vi "KenbakFront.vi"() -> ()   [LabVIEW 2012]
panel:
  in  "Data":u8 format="%08b"
  out "Kdec":u8
  in  "Read":bool
  in  "Store":bool
  in  "AddressDec":u8
  in  "Inputs":T1
  in  "Wait (ms)":u32
  out "Instruction Specific":T2
  out "Adder":T3
  out "Clocks And Memory":T4
  out "W_reg":T5
  out "L_reg":T6
  out "T_reg":T7
  out "Mem":cluster{"MemLo":u8, "MemHi":u8, "Carry?":bool} {"MemHi" format="%x"; "MemLo" format="%x"}
  out "I_reg":T8
  out "States":T9
  out "Input":bool
  out "Run":bool
  out "Memory":bool
  out "Address":bool
  out "K_reg":T10
  out "Cycles/sec":i32
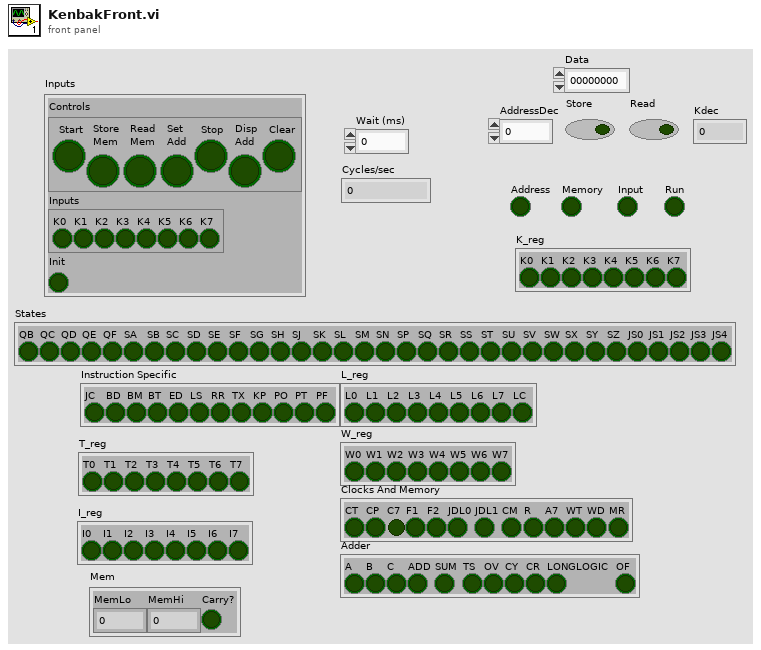
[diagram p1: front panel]
types:
  T1 = cluster{"Controls":cluster{"Start":bool, "Store\nMem":bool, "Read\nMem":bool, "Set\nAdd":bool, "Stop":bool, "Disp\nAdd":bool, "Clear":bool}, "Inputs":cluster{"K0":bool, "K1":bool, "K2":bool, "K3":bool, "K4":bool, "K5":bool, "K6":bool, "K7":bool}, "Init":bool}
  T2 = cluster{"JC":bool, "BD":bool, "BM":bool, "BT":bool, "ED":bool, "LS":bool, "RR":bool, "TX":bool, "KP":bool, "PO":bool, "PT":bool, "PF":bool}
  T3 = cluster{"A":bool, "B":bool, "C":bool, "ADD":bool, "SUM":bool, "TS":bool, "OV":bool, "CY":bool, "CR":bool, "LONGLOGIC":bool, "OF":bool}
  T4 = cluster{"CT":bool, "CP":bool, "C7":bool, "F1":bool, "F2":bool, "JDL0":bool, "JDL1":bool, "CM":bool, "R":bool, "A7":bool, "WT":bool, "WD":bool, "MR":bool}
  T5 = cluster{"W0":bool, "W1":bool, "W2":bool, "W3":bool, "W4":bool, "W5":bool, "W6":bool, "W7":bool}
  T6 = cluster{"L0":bool, "L1":bool, "L2":bool, "L3":bool, "L4":bool, "L5":bool, "L6":bool, "L7":bool, "LC":bool}
  T7 = cluster{"T0":bool, "T1":bool, "T2":bool, "T3":bool, "T4":bool, "T5":bool, "T6":bool, "T7":bool}
  T8 = cluster{"I0":bool, "I1":bool, "I2":bool, "I3":bool, "I4":bool, "I5":bool, "I6":bool, "I7":bool}
  T9 = cluster{"QB":bool, "QC":bool, "QD":bool, "QE":bool, "QF":bool, "SA":bool, "SB":bool, "SC":bool, "SD":bool, "SE":bool, "SF":bool, "SG":bool, "SH":bool, "SJ":bool, "SK":bool, "SL":bool, "SM":bool, "SN":bool, "SP":bool, "SQ":bool, "SR":bool, "SS":bool, "ST":bool, "SU":bool, "SV":bool, "SW":bool, "SX":bool, "SY":bool, "SZ":bool, "JS0":bool, "JS1":bool, "JS2":bool, "JS3":bool, "JS4":bool}
  T10 = cluster{"K0":bool, "K1":bool, "K2":bool, "K3":bool, "K4":bool, "K5":bool, "K6":bool, "K7":bool}
  T11 = cluster{"[0]":bool, "[1]":bool, "[2]":bool, "[3]":bool, "[4]":bool, "[5]":bool, "[6]":bool, "[7]":bool}
  T12 = cluster{"GO":bool, "EN":bool, "DD":bool, "EA":bool, "HT":bool, "DA":bool, "CL":bool, "ADD":bool, "MEM":bool, "RUN":bool, "INPUT":bool, "X1":bool, "X2":bool, "X3":bool, "X4":bool, "BU":bool, "KS":bool, "FT":bool}
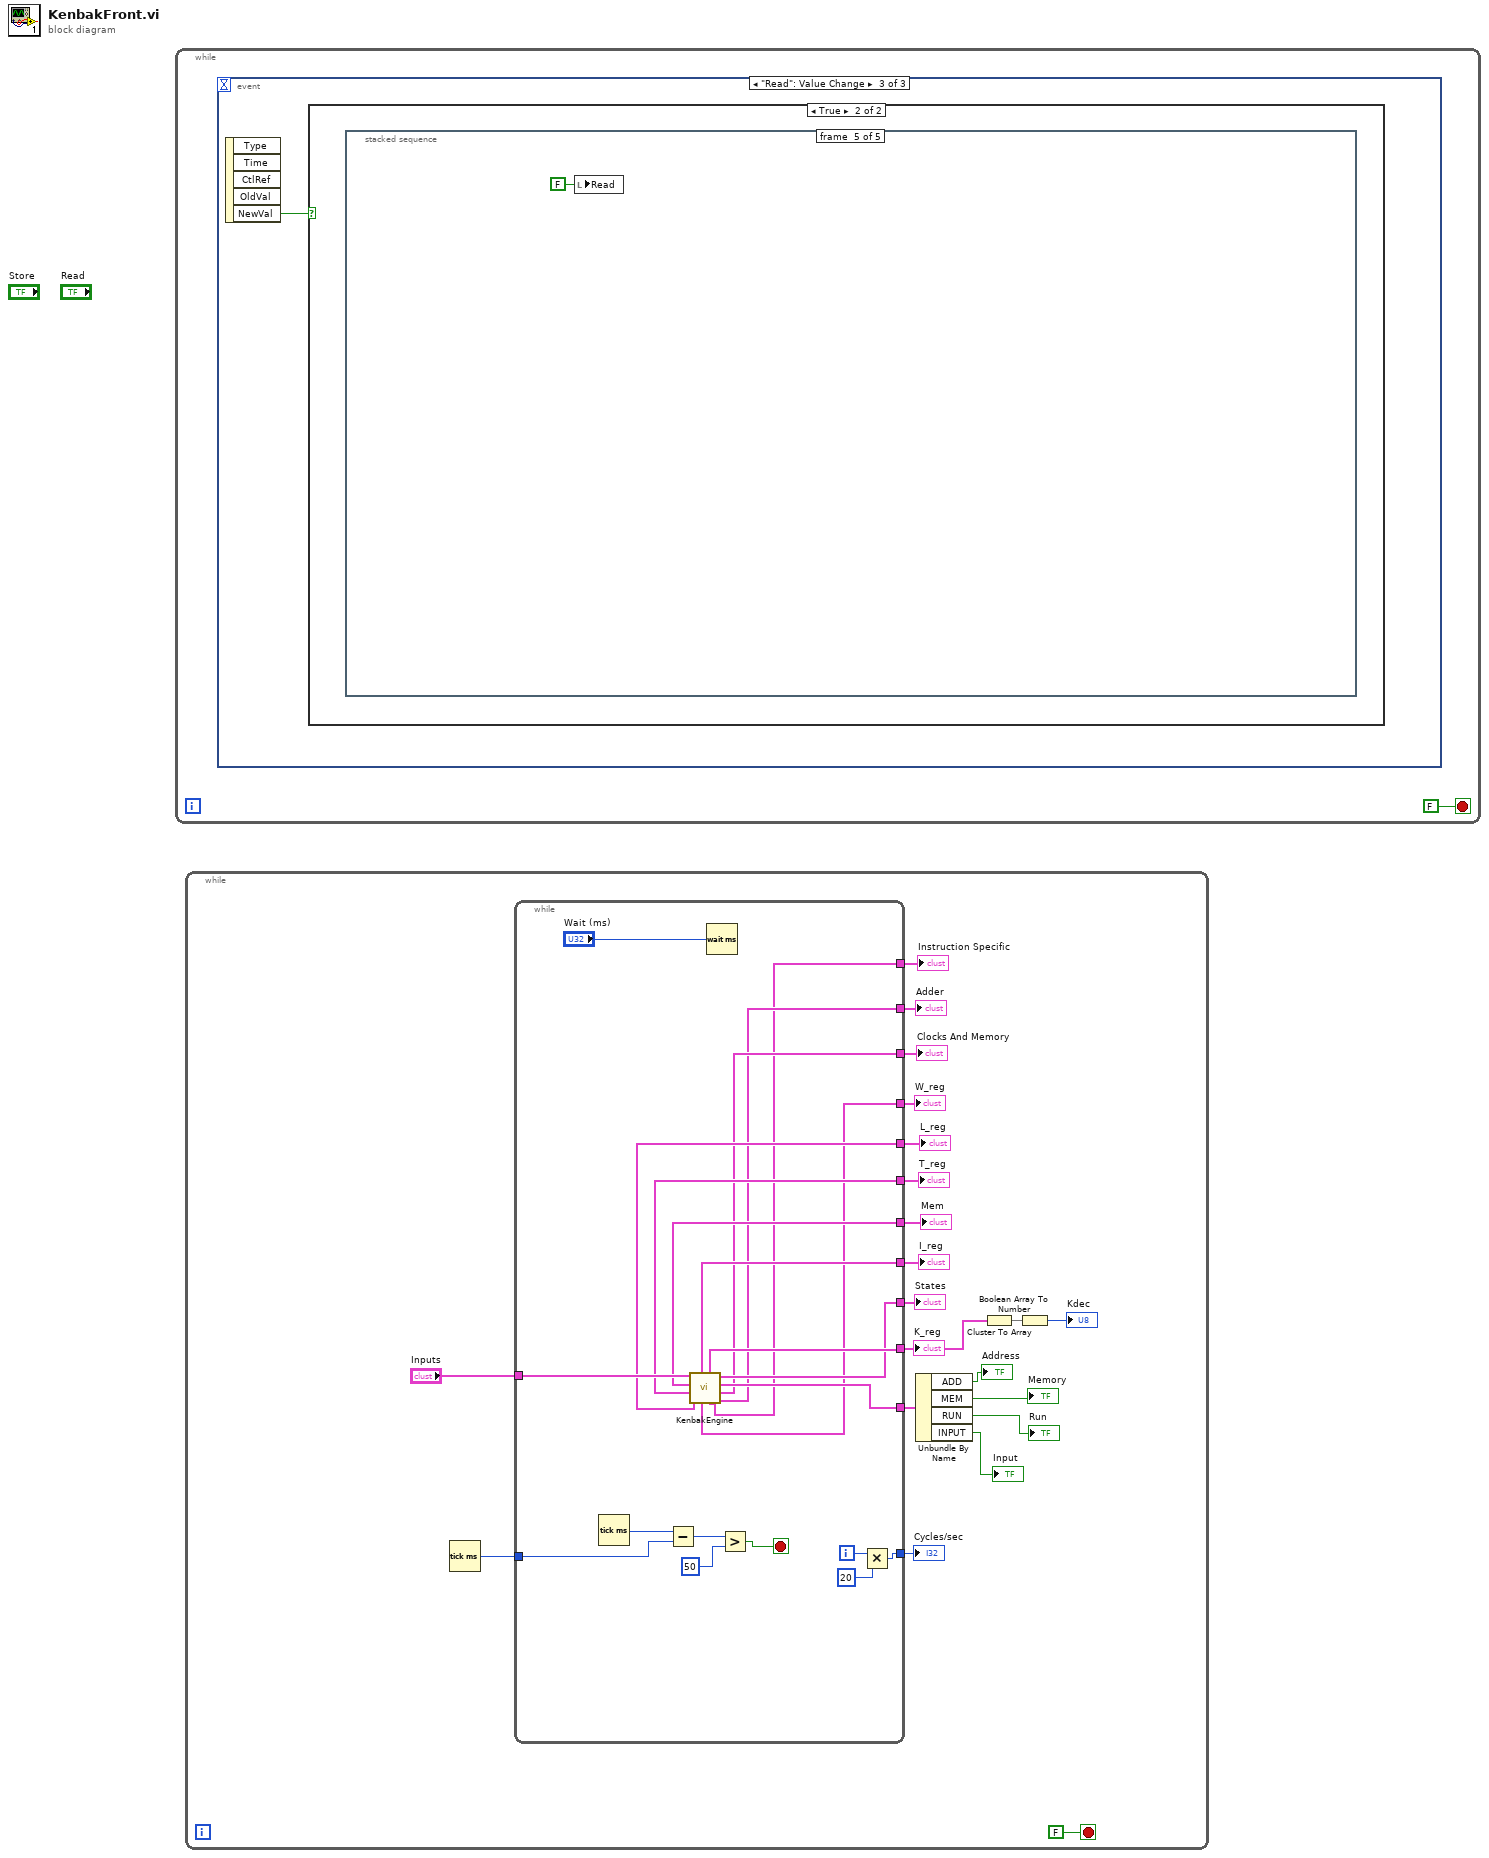
[diagram p0: block diagram]
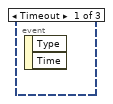
[diagram p2: hidden frame]
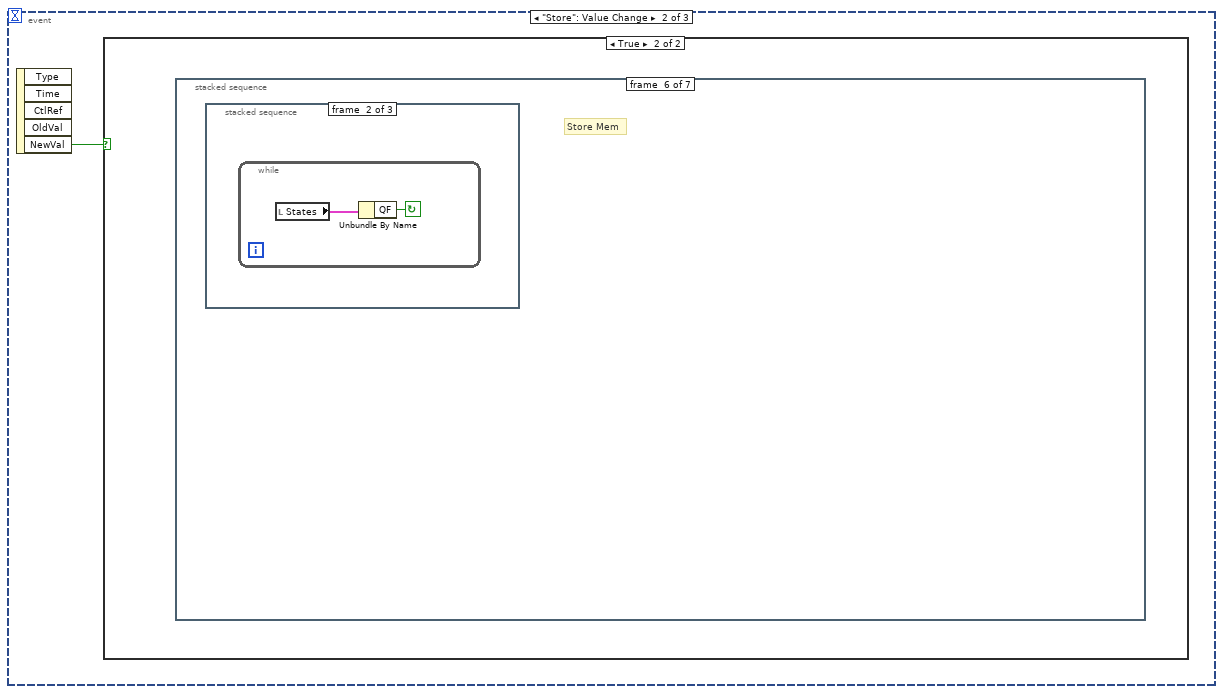
[diagram p3: hidden frame]
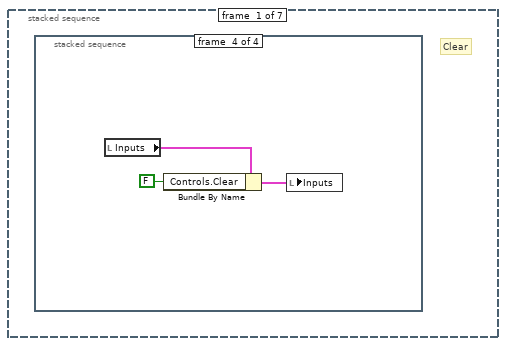
[diagram p5: hidden frame]
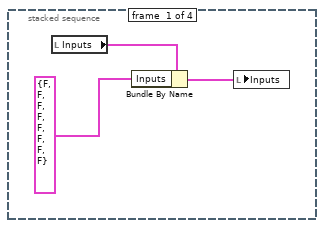
[diagram p6: hidden frame]
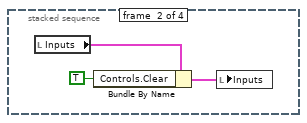
[diagram p7: hidden frame]
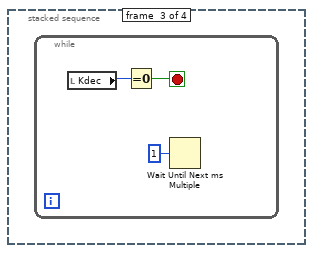
[diagram p8: hidden frame]
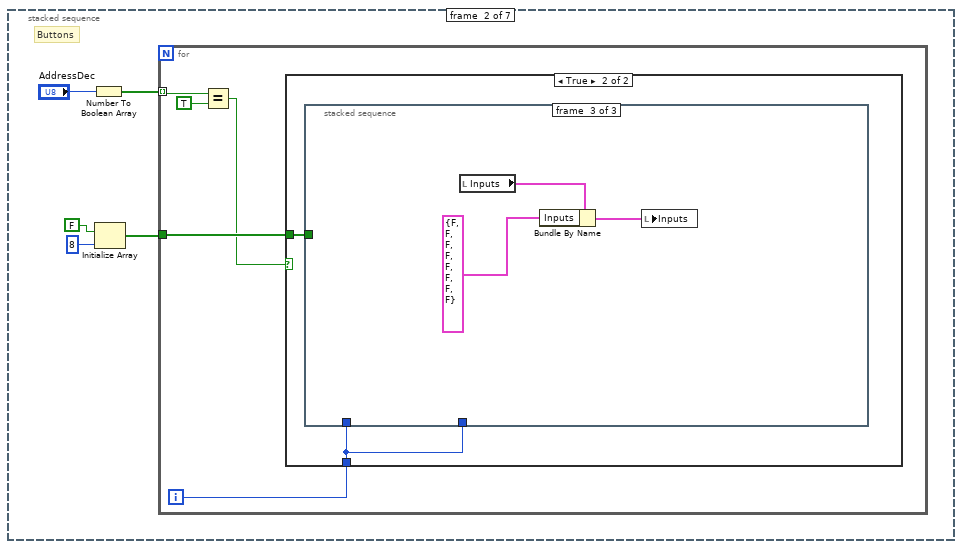
[diagram p9: hidden frame]
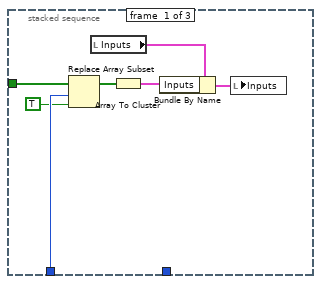
[diagram p11: hidden frame]
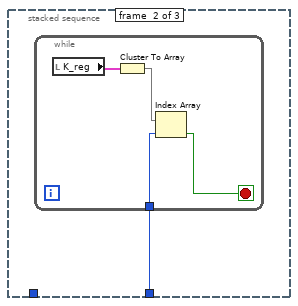
[diagram p12: hidden frame]
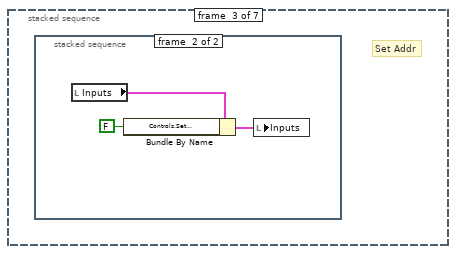
[diagram p13: hidden frame]
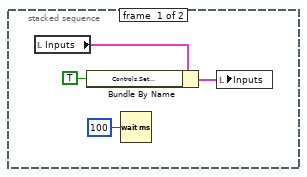
[diagram p14: hidden frame]
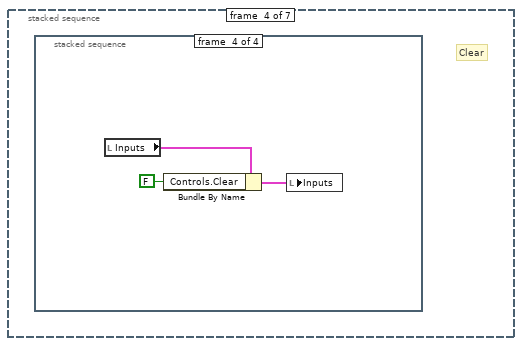
[diagram p15: hidden frame]
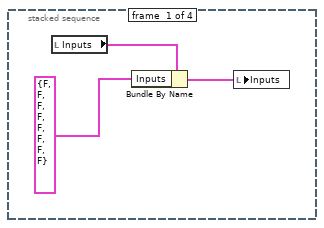
[diagram p16: hidden frame]
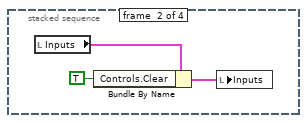
[diagram p17: hidden frame]
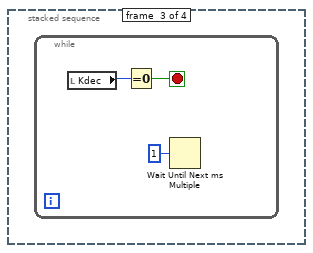
[diagram p18: hidden frame]
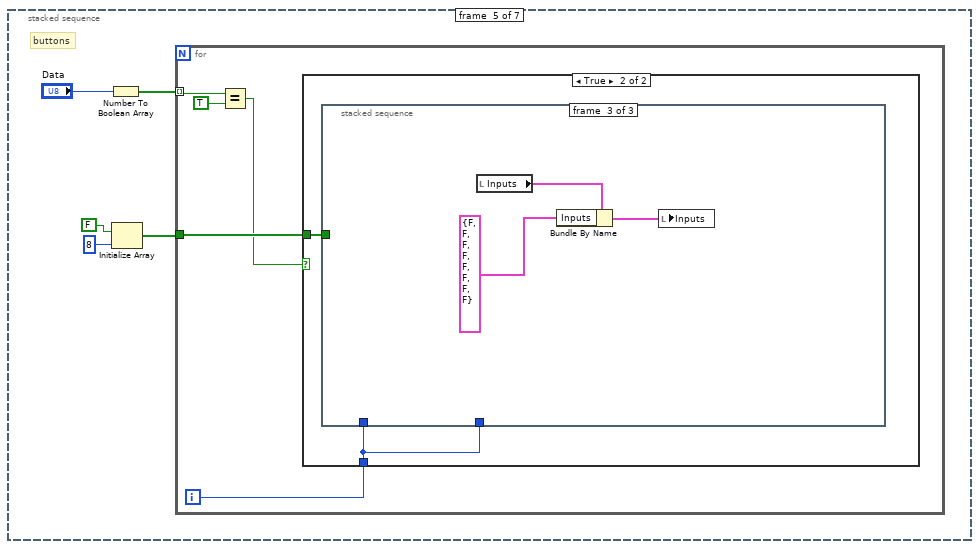
[diagram p19: hidden frame]
diagram:
  n1 = while {
    stop <- FALSE stop-if-true
    n2 = event shown="[2] \"Read\": Value Change" {
      selector: _ -> [_ _ _]
      dyn-events: _ -> [_ _ _]
      timeout: _ -> [_ _ _]
      event Timeout {
        n3 = event-data() -> ()  [unwired: 1 in, 2 out]
      }
      event "Store": Value Change {
        n4 = event-data() -> ("NewVal"=w2:bool)  [unwired: 1 in, 4 out]
        n5 = case shown="True" w2 {
          frame False {
          }
          frame True {
            n6 = stacked-sequence {
              frame #0 {
                # "Clear"
                n7 = stacked-sequence {
                  frame #0 {
                    n8 = local read "Inputs"() -> (w3:T1)
                    n9 = Bundle By Name(cluster=w3, "Inputs"=T10 {"K0"=FALSE, "K1"=FALSE, "K2"=FALSE, "K3"=FALSE, "K4"=FALSE, "K5"=FALSE, "K6"=FALSE, "K7"=FALSE}) -> (w4:T1)
                    n10 = local write "Inputs"(w4) -> ()
                  }
                  frame #1 {
                    n11 = local read "Inputs"() -> (w6:T1)
                    n12 = Bundle By Name(cluster=w6, "Controls.Clear"=TRUE) -> (w7:T1)
                    n13 = local write "Inputs"(w7) -> ()
                  }
                  frame #2 {
                    n14 = while {
                      stop <- w10 stop-if-true
                      n15 = local read "Kdec"() -> (w11:u8)
                      n16 = Equal To 0?(x=w11) -> (x = 0?=w10:bool)
                      n17 = Wait Until Next ms Multiple(millisecond multiple=u32 1) -> ()  [unwired: 1 out]
                    }
                  }
                  frame #3 {
                    n18 = local read "Inputs"() -> (w12:T1)
                    n19 = Bundle By Name(cluster=w12, "Controls.Clear"=FALSE) -> (w13:T1)
                    n20 = local write "Inputs"(w13) -> ()
                  }
                }
              }
              frame #1 {
                # "Buttons"
                n21 = Number To Boolean Array(number="AddressDec") -> (Boolean array=w18:bool[])
                n22 = Initialize Array(FALSE ("new element/subarray"), 8 ("dimension size")) -> (w15:bool[])
                n23 = for {
                  tunnel: w18 -> [w24] mode=indexing
                  tunnel: w15 -> [w21]
                  i -> [w22]
                  n24 = Equal?(x=w24, y=TRUE) -> (x = y?=w20:bool)
                  n25 = case shown="True" w20 {
                    tunnel: w22 -> [_ w25]
                    tunnel: w21 -> [_ w26]
                    frame False {
                    }
                    frame True {
                      n26 = stacked-sequence {
                        tunnel: w25 -> [w32 _ _]
                        tunnel: w26 -> [w29 _ _]
                        tunnel: w25 -> [_ w34 _]
                        frame #0 {
                          n27 = Replace Array Subset(array=w29, new element=TRUE ("new element/subarray"), index=w32) -> (w28:bool[])
                          n28 = local read "Inputs"() -> (w30:T1)
                          n29 = Array To Cluster(array=w28) -> (cluster=w27:T11)
                          n30 = Bundle By Name(cluster=w30, "Inputs"=w27) -> (w33:T1)
                          n31 = local write "Inputs"(w33) -> ()
                        }
                        frame #1 {
                          n32 = while {
                            tunnel: w34 -> [w36]
                            stop <- w35 stop-if-true
                            n33 = local read "K_reg"() -> (w38:T10)
                            n34 = Cluster To Array(cluster=w38) -> (array=w37:bool[])
                            n35 = Index Array(array=w37, index=w36) -> (element=w35:bool)
                          }
                        }
                        frame #2 {
                          n36 = local read "Inputs"() -> (w41:T1)
                          n37 = Bundle By Name(cluster=w41, "Inputs"=T10 {"K0"=FALSE, "K1"=FALSE, "K2"=FALSE, "K3"=FALSE, "K4"=FALSE, "K5"=FALSE, "K6"=FALSE, "K7"=FALSE}) -> (w40:T1)
                          n38 = local write "Inputs"(w40) -> ()
                        }
                      }
                    }
                  }
                }
              }
              frame #2 {
                # "Set Addr"
                n39 = stacked-sequence {
                  frame #0 {
                    n40 = local read "Inputs"() -> (w43:T1)
                    n41 = Bundle By Name(cluster=w43, "Controls.Set\nAdd"=TRUE ("Controls.Set\nAdd")) -> (w44:T1)
                    n42 = Wait (ms)(milliseconds to wait=u32 100) -> ()  [unwired: 1 out]
                    n43 = local write "Inputs"(w44) -> ()
                  }
                  frame #1 {
                    n44 = local read "Inputs"() -> (w46:T1)
                    n45 = Bundle By Name(cluster=w46, "Controls.Set\nAdd"=FALSE ("Controls.Set\nAdd")) -> (w47:T1)
                    n46 = local write "Inputs"(w47) -> ()
                  }
                }
              }
              frame #3 {
                # "Clear"
                n47 = stacked-sequence {
                  frame #0 {
                    n48 = local read "Inputs"() -> (w49:T1)
                    n49 = Bundle By Name(cluster=w49, "Inputs"=T10 {"K0"=FALSE, "K1"=FALSE, "K2"=FALSE, "K3"=FALSE, "K4"=FALSE, "K5"=FALSE, "K6"=FALSE, "K7"=FALSE}) -> (w50:T1)
                    n50 = local write "Inputs"(w50) -> ()
                  }
                  frame #1 {
                    n51 = local read "Inputs"() -> (w52:T1)
                    n52 = Bundle By Name(cluster=w52, "Controls.Clear"=TRUE) -> (w53:T1)
                    n53 = local write "Inputs"(w53) -> ()
                  }
                  frame #2 {
                    n54 = while {
                      stop <- w56 stop-if-true
                      n55 = local read "Kdec"() -> (w57:u8)
                      n56 = Equal To 0?(x=w57) -> (x = 0?=w56:bool)
                      n57 = Wait Until Next ms Multiple(millisecond multiple=u32 1) -> ()  [unwired: 1 out]
                    }
                  }
                  frame #3 {
                    n58 = local read "Inputs"() -> (w58:T1)
                    n59 = Bundle By Name(cluster=w58, "Controls.Clear"=FALSE) -> (w59:T1)
                    n60 = local write "Inputs"(w59) -> ()
                  }
                }
              }
              frame #4 {
                # "buttons"
                n61 = Number To Boolean Array(number="Data") -> (Boolean array=w65:bool[])
                n62 = Initialize Array(FALSE ("new element/subarray"), 8 ("dimension size")) -> (w62:bool[])
                n63 = for {
                  tunnel: w65 -> [w70] mode=indexing
                  tunnel: w62 -> [w67]
                  i -> [w68]
                  n64 = Equal?(x=w70, y=TRUE) -> (x = y?=w66:bool)
                  n65 = case shown="True" w66 {
                    tunnel: w68 -> [_ w71]
                    tunnel: w67 -> [_ w72]
                    frame False {
                    }
                    frame True {
                      n66 = stacked-sequence {
                        tunnel: w71 -> [w78 _ _]
                        tunnel: w72 -> [w75 _ _]
                        tunnel: w71 -> [_ w80 _]
                        frame #0 {
                          n67 = Replace Array Subset(array=w75, new element=TRUE ("new element/subarray"), index=w78) -> (w74:bool[])
                          n68 = local read "Inputs"() -> (w76:T1)
                          n69 = Array To Cluster(array=w74) -> (cluster=w73:T11)
                          n70 = Bundle By Name(cluster=w76, "Inputs"=w73) -> (w79:T1)
                          n71 = local write "Inputs"(w79) -> ()
                        }
                        frame #1 {
                          n72 = while {
                            tunnel: w80 -> [w82]
                            stop <- w81 stop-if-true
                            n73 = local read "K_reg"() -> (w84:T10)
                            n74 = Cluster To Array(cluster=w84) -> (array=w83:bool[])
                            n75 = Index Array(array=w83, index=w82) -> (element=w81:bool)
                          }
                        }
                        frame #2 {
                          n76 = local read "Inputs"() -> (w87:T1)
                          n77 = Bundle By Name(cluster=w87, "Inputs"=T10 {"K0"=FALSE, "K1"=FALSE, "K2"=FALSE, "K3"=FALSE, "K4"=FALSE, "K5"=FALSE, "K6"=FALSE, "K7"=FALSE}) -> (w86:T1)
                          n78 = local write "Inputs"(w86) -> ()
                        }
                      }
                    }
                  }
                }
              }
              frame #5 {
                # "Store Mem"
                n79 = stacked-sequence {
                  frame #0 {
                    n80 = local read "Inputs"() -> (w88:T1)
                    n81 = Bundle By Name(cluster=w88, "Controls.Store\nMem"=TRUE ("Controls.Store\nMem")) -> (w89:T1)
                    n82 = local write "Inputs"(w89) -> ()
                  }
                  frame #1 {
                    n83 = while {
                      stop <- w91 continue-if-true
                      n84 = local read "States"() -> (w92:T9)
                      n85 = Unbundle By Name(w92) -> ("QF"=w91:bool)
                    }
                  }
                  frame #2 {
                    n86 = local read "Inputs"() -> (w93:T1)
                    n87 = Bundle By Name(cluster=w93, "Controls.Store\nMem"=FALSE ("Controls.Store\nMem")) -> (w94:T1)
                    n88 = local write "Inputs"(w94) -> ()
                  }
                }
              }
              frame #6 {
                n89 = local write "Store"(FALSE ("Store")) -> ()
              }
            }
          }
        }
      }
      event "Read": Value Change {
        n90 = event-data() -> ("NewVal"=w97:bool)  [unwired: 1 in, 4 out]
        n91 = case shown="True" w97 {
          frame False {
          }
          frame True {
            n92 = stacked-sequence {
              frame #0 {
                n93 = stacked-sequence {
                  frame #0 {
                    n94 = local read "Inputs"() -> (w98:T1)
                    n95 = Bundle By Name(cluster=w98, "Inputs"=T10 {"K0"=FALSE, "K1"=FALSE, "K2"=FALSE, "K3"=FALSE, "K4"=FALSE, "K5"=FALSE, "K6"=FALSE, "K7"=FALSE}) -> (w99:T1)
                    n96 = local write "Inputs"(w99) -> ()
                  }
                  frame #1 {
                    n97 = local read "Inputs"() -> (w101:T1)
                    n98 = Bundle By Name(cluster=w101, "Controls.Clear"=TRUE) -> (w102:T1)
                    n99 = local write "Inputs"(w102) -> ()
                  }
                  frame #2 {
                    n100 = while {
                      stop <- w105 stop-if-true
                      n101 = local read "Kdec"() -> (w106:u8)
                      n102 = Equal To 0?(x=w106) -> (x = 0?=w105:bool)
                      n103 = Wait Until Next ms Multiple(millisecond multiple=u32 1) -> ()  [unwired: 1 out]
                    }
                  }
                  frame #3 {
                    n104 = local read "Inputs"() -> (w107:T1)
                    n105 = Bundle By Name(cluster=w107, "Controls.Clear"=FALSE) -> (w108:T1)
                    n106 = local write "Inputs"(w108) -> ()
                  }
                }
              }
              frame #1 {
                # "Buttons"
                n107 = local read "AddressDec"() -> (w114:u8)
                n108 = Number To Boolean Array(number=w114) -> (Boolean array=w113:bool[])
                n109 = Initialize Array(FALSE ("new element/subarray"), 8 ("dimension size")) -> (w110:bool[])
                n110 = for {
                  tunnel: w113 -> [w119] mode=indexing
                  tunnel: w110 -> [w116]
                  i -> [w117]
                  n111 = Equal?(x=w119, y=TRUE) -> (x = y?=w115:bool)
                  n112 = case shown="True" w115 {
                    tunnel: w117 -> [_ w120]
                    tunnel: w116 -> [_ w121]
                    frame False {
                    }
                    frame True {
                      n113 = stacked-sequence {
                        tunnel: w120 -> [w127 _ _]
                        tunnel: w121 -> [w124 _ _]
                        tunnel: w120 -> [_ w129 _]
                        frame #0 {
                          n114 = Replace Array Subset(array=w124, new element=TRUE ("new element/subarray"), index=w127) -> (w123:bool[])
                          n115 = local read "Inputs"() -> (w125:T1)
                          n116 = Array To Cluster(array=w123) -> (cluster=w122:T11)
                          n117 = Bundle By Name(cluster=w125, "Inputs"=w122) -> (w128:T1)
                          n118 = local write "Inputs"(w128) -> ()
                        }
                        frame #1 {
                          n119 = while {
                            tunnel: w129 -> [w131]
                            stop <- w130 stop-if-true
                            n120 = local read "K_reg"() -> (w133:T10)
                            n121 = Cluster To Array(cluster=w133) -> (array=w132:bool[])
                            n122 = Index Array(array=w132, index=w131) -> (element=w130:bool)
                          }
                        }
                        frame #2 {
                          n123 = local read "Inputs"() -> (w136:T1)
                          n124 = Bundle By Name(cluster=w136, "Inputs"=T10 {"K0"=FALSE, "K1"=FALSE, "K2"=FALSE, "K3"=FALSE, "K4"=FALSE, "K5"=FALSE, "K6"=FALSE, "K7"=FALSE}) -> (w135:T1)
                          n125 = local write "Inputs"(w135) -> ()
                        }
                      }
                    }
                  }
                }
              }
              frame #2 {
                n126 = stacked-sequence {
                  frame #0 {
                    n127 = local read "Inputs"() -> (w138:T1)
                    n128 = Bundle By Name(cluster=w138, "Controls.Set\nAdd"=TRUE ("Controls.Set\nAdd")) -> (w139:T1)
                    n129 = Wait (ms)(milliseconds to wait=u32 100) -> ()  [unwired: 1 out]
                    n130 = local write "Inputs"(w139) -> ()
                  }
                  frame #1 {
                    n131 = local read "Inputs"() -> (w141:T1)
                    n132 = Bundle By Name(cluster=w141, "Controls.Set\nAdd"=FALSE ("Controls.Set\nAdd")) -> (w142:T1)
                    n133 = local write "Inputs"(w142) -> ()
                  }
                }
              }
              frame #3 {
                n134 = stacked-sequence {
                  frame #0 {
                    n135 = local read "Inputs"() -> (w144:T1)
                    n136 = Bundle By Name(cluster=w144, "Controls.Read\nMem"=TRUE ("Controls.Store\nMem")) -> (w145:T1)
                    n137 = local write "Inputs"(w145) -> ()
                  }
                  frame #1 {
                    n138 = while {
                      stop <- w147 continue-if-true
                      n139 = local read "States"() -> (w148:T9)
                      n140 = Unbundle By Name(w148) -> ("QF"=w147:bool)
                    }
                  }
                  frame #2 {
                    n141 = local read "Inputs"() -> (w149:T1)
                    n142 = Bundle By Name(cluster=w149, "Controls.Read\nMem"=FALSE ("Controls.Store\nMem")) -> (w150:T1)
                    n143 = local write "Inputs"(w150) -> ()
                  }
                }
              }
              frame #4 {
                n144 = local write "Read"(FALSE ("Read")) -> ()
              }
            }
          }
        }
      }
    }
  }
  n145 = while {
    stop <- FALSE stop-if-true
    n146 = Tick Count (ms)() -> (millisecond timer value=w173:u32)
    n147 = while {
      tunnel: w173 -> [w193]
      tunnel: [w187] -> w172
      tunnel: "Inputs" -> [w186]
      tunnel: [w185] -> w155
      tunnel: [w184] -> w166
      tunnel: [w183] -> w165
      tunnel: [w182] -> w164
      tunnel: [w181] -> w163
      tunnel: [w180] -> w162
      tunnel: [w179] -> w161
      tunnel: [w178] -> w160
      tunnel: [w177] -> w159
      tunnel: [w176] -> w158
      tunnel: [w175] -> w157
      i -> [w189]
      stop <- w190 stop-if-true
      n148 = Tick Count (ms)() -> (millisecond timer value=w194:u32)
      n149 = Subtract(x=w194, y=w193) -> (x-y=w192:u32)
      n150 = call "KenbakEngine.vi"("Inputs"=w186) -> ("Adder"=w176:T3, "Clocks And Memory"=w177:T4, "Control\nSignals"=w184:T12, "States"=w183:T9, "Instruction Specific"=w175:T2, "K_reg"=w185:T10, "W_reg"=w178:T5, "I_reg"=w182:T8, "L_reg"=w179:T6, "T_reg"=w180:T7, "Memory"=w181:cluster{"MemLo":u8, "MemHi":u8, "Carry?":bool})
      n151 = Wait (ms)(milliseconds to wait="Wait (ms)") -> ()  [unwired: 1 out]
      n152 = Greater?(x=w192, y=u32 50) -> (0:w190:bool)
      n153 = Multiply(x=w189, y=20) -> (x*y=w187:i32)
    }
    "Cycles/sec" <- w172
    "K_reg" <- w155
    "States" <- w165
    "I_reg" <- w164
    "Mem" <- w163
    "T_reg" <- w162
    "L_reg" <- w161
    "W_reg" <- w160
    "Clocks And Memory" <- w159
    "Adder" <- w158
    "Instruction Specific" <- w157
    n154 = Unbundle By Name(w166) -> ("ADD"=→"Address":bool, "MEM"=→"Memory":bool, "RUN"=→"Run":bool, "INPUT"=→"Input":bool)
    n155 = Cluster To Array(cluster=w155) -> (array=w154:bool[])
    n156 = Boolean Array To Number(Boolean array=w154) -> (number=→"Kdec":u32)
  }
